vi "Write Pressure Servo Center Point.vi"(10 "Pressure Servo Center Point":dbl[unit], 11 "Model in":refnum<class "Model.lvclass">) -> (3 "Model out":refnum<class "Model.lvclass">)   [LabVIEW 2015, in "Model.lvclass"]
uses:
  Model.lvclass
  Model.lvclass/Model.ctl
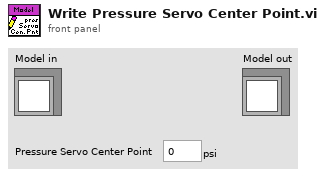
[diagram p1: front panel]
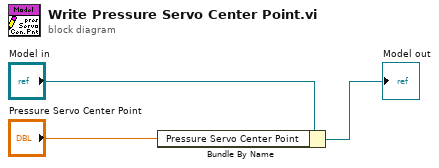
[diagram p0: block diagram]
diagram:
  n1 = Bundle By Name(cluster="Model in", "Pressure Servo Center Point"="Pressure Servo Center Point") -> (→"Model out":refnum<class "Model.lvclass">)
